vi "Write Abstract Message Msg.vi"(10 "Nested Actor.lvlib:Abstract Message Msg.lvclass":refnum<class "Abstract Message Msg.lvclass">, 11 "Nested Actor in":refnum<class "Nested Actor.lvclass">) -> (3 "Nested Actor out":refnum<class "Nested Actor.lvclass">)   [LabVIEW 2020, in "Nested Actor.lvlib" / "Nested Actor.lvclass"]
uses:
  Nested Actor.lvclass
  Nested Actor Messages/Abstract Message Msg/Abstract Message Msg.lvclass
  Nested Actor.lvclass/Nested Actor.ctl
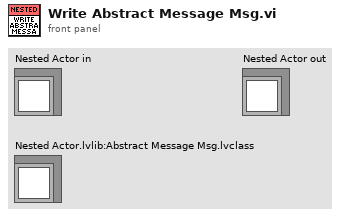
[diagram p1: front panel]
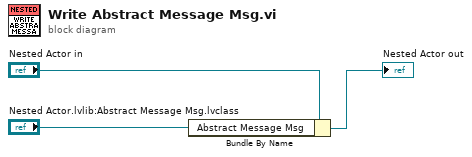
[diagram p0: block diagram]
diagram:
  n1 = Bundle By Name(cluster="Nested Actor in", "Abstract Message Msg"="Nested Actor.lvlib:Abstract Message Msg.lvclass") -> (→"Nested Actor out":refnum<class "Nested Actor.lvclass">)
